vi "诊断标定4.vi"(8 "CAN端口":u16(ring), 9 "设备索引号":u16(ring), 10 "CAN卡类型":u32(ring)=4) -> ()   [LabVIEW 2013] (continued)
      n52 = property class="MCListbox (严格)"(reference=w20, "ItemNames"=w19) -> ()  [unwired: 1 in, 2 out]
      n53 = property on="全部读取" class="Bool (严格)"("Visible"=w95) -> ()  [unwired: 2 in, 2 out]
      n54 = Insert Into Array(array=w61, new element #1=w60, new element #2=w59, new element #3=w58, new element #4=w57, new element #5=w56) -> (w55:bool[])  [unwired: 1 in]
      n55 = local write "主从选择"(enum32{"主板", "从板"}."主板" ("主从选择")) -> ()
      n56 = And Array Elements(Boolean array=w55) -> (logical AND=w94:bool)
      n57 = property on="全部写入" class="Bool (严格)"("DisabledEnum"=2) -> ()  [unwired: 2 in, 2 out]
      n58 = local write "布尔"(w24) -> ()
      n59 = property on="全部写入" class="Bool (严格)"("Visible"=w94) -> ()  [unwired: 2 in, 2 out]
      n60 = local write "等级 2"(T13."从板信息" ("等级 2")) -> ()
      n61 = control-ref of="结果"() -> (w31:refnum<vi>)
      n62 = control-ref of="结果"() -> (w28:refnum<vi>)
      n63 = control-ref of="项目信息"() -> (w29:refnum<vi>)
      n64 = global write "EV05全局变量1.vi" "授权功能"(w25) -> ()
      n65 = local write "整车CAN测试"(w25) -> ()
      n66 = local write "判定2"(w25) -> ()
      n67 = local write "停止"(w25) -> ()
      n68 = local write "控制1"(w25) -> ()
      n69 = local write "消除"(w25) -> ()
      n70 = local write "继电器超时处理"(w25) -> ()
      n71 = local write "1 6"(w25) -> ()
      n72 = local write "1 7"(w25) -> ()
      n73 = local write "1 8"(w25) -> ()
      n74 = local write "1 9"(w25) -> ()
      n75 = local write "1 10"(w25) -> ()
      n76 = local write "1 2"(w25) -> ()
      n77 = local write "1 3"(w25) -> ()
      n78 = local write "1 4"(w25) -> ()
      n79 = local write "1 5"(w25) -> ()
      n80 = local write "1 11"(w25) -> ()
      n81 = local write "强制停止"(w25) -> ()
      n82 = for {
        N: 150 -> [_]
        tunnel: w31 -> [w123]
        i -> [w121]
        n83 = Bundle(w121, 0) -> (w119:cluster{i32, i32})  [unwired: 1 out]
        n84 = property class="MCListbox (严格)"(reference=w123, "ActiveCell"=w119, "CellBG"=u32 16448250) -> ()  [unwired: 1 in, 2 out]
        n85 = Wait Until Next ms Multiple(millisecond multiple=u32 1 ("毫秒倍数")) -> ()  [unwired: 1 out]
      }
      n86 = for {
        N: 150 -> [_]
        tunnel: w29 -> [w117]
        i -> [w116]
        n87 = Bundle(w116, 0) -> (w114:cluster{i32, i32})  [unwired: 1 out]
        n88 = property class="Tbl (严格)"(reference=w117, "Active Cell"=w114, "Cell BG Color"=u32 16448250) -> ()  [unwired: 1 in, 2 out]
        n89 = Wait Until Next ms Multiple(millisecond multiple=u32 1 ("毫秒倍数")) -> ()  [unwired: 1 out]
      }
      n90 = for {
        N: 150 -> [_]
        tunnel: w28 -> [w129]
        i -> [w127]
        n91 = Bundle(w127, 0) -> (w125:cluster{i32, i32})  [unwired: 1 out]
        n92 = property class="MCListbox (严格)"(reference=w129, "ActiveCell"=w125, "CellBG"=u32 16448250) -> ()  [unwired: 1 in, 2 out]
        n93 = Wait Until Next ms Multiple(millisecond multiple=u32 1 ("毫秒倍数")) -> ()  [unwired: 1 out]
      }
      n94 = stacked-sequence {
        tunnel: [w96 _] -> w23
        frame #0 {
          w103 = u8 0 items=["Normal", "Listen Only"] ("工作方式")
          w102 = u8 1 items=["Dual Filter", "Single Filter"] ("滤波方式")
          n95 = local read "设备索引号"() -> (w98:u16)
          n96 = local read "CAN卡类型"() -> (w97:u32)
          n97 = local read "CAN端口"() -> (w99:u16)
          n98 = call "CAN_Init-8.6.vi"("CAN卡类型"=w97, "设备索引号"=w98, "CAN端口"=w99, "操作类型"=enum16{"初始化CAN", "关闭CAN"}."初始化CAN", "滤波方式"=w102, "Accept Code"=u32 3221225472, "簇"=T20 {"打开CAN"=FALSE, "初始化CAN"=TRUE, "开始CAN"=TRUE, "重启"=FALSE, "关闭CAN"=FALSE}, "Mask Code"=u32 1073741823 ("Accept Code"), "工作方式"=w103, "是否滤波"=TRUE, "滤波选择"=T19 {"fiter_mode"=1, "fiter_endid"=402653184, "fiter_startid"=419430399}) -> ("error out"=w96:errorcluster)  [unwired: 3 in, 5 out]
        }
        frame #1 {
          n99 = local read "设备索引号"() -> (w109:u16)
          n100 = local read "CAN卡类型"() -> (w108:u32)
          n101 = local read "CAN端口"() -> (w110:u16)
          n102 = dll-call lib="PTH1Aabs EEV05EV05监控上位机-EV05EV05data\nusbcan.dll" fn="VCI_ClearBuffer"("DeviceType"=w108, "DeviceInd"=w109, "CANInd"=w110) -> (error out=w111:errorcluster)  [unwired: 4 in, 4 out]
          n103 = call <vilib>:"Clear Errors.vi"("error in (no error)"=w111) -> ()  [unwired: 6 in, 1 out]
        }
      }
      n104 = property on="保存版本信息" class="Bool (严格)"("Visible"=w25) -> ()  [unwired: 2 in, 2 out]
      n105 = local write "正级继电器"(w25) -> ()
      n106 = local write "负级继电器"(w25) -> ()
      n107 = local write "预充电继电器"(w25) -> ()
      n108 = local write "加热继电器"(w25) -> ()
      n109 = local write "充电继电器"(w25) -> ()
      n110 = local write "风机继电器"(w25) -> ()
      n111 = local write "加热继电器"(w25) -> ()
      n112 = local write "风机继电器"(w25) -> ()
      n113 = local write "DO1"(w25) -> ()
      n114 = local write "DO2"(w25) -> ()
      n115 = local write "DO1 2"(w25) -> ()
      n116 = local write "正级继电器 12"(w25) -> ()
      n117 = local write "正级继电器 2"(w25) -> ()
      n118 = local write "正级继电器 3"(w25) -> ()
      n119 = local write "正级继电器 4"(w25) -> ()
      n120 = local write "正级继电器 5"(w25) -> ()
      n121 = local write "正级继电器 6"(w25) -> ()
      n122 = local write "正级继电器 7"(w25) -> ()
      n123 = local write "正级继电器 8"(w25) -> ()
      n124 = local write "正级继电器 9"(w25) -> ()
      n125 = local write "正级继电器 10"(w25) -> ()
      n126 = local write "正级继电器 11"(w25) -> ()
      "电池故障" <- string[][] []
      "模块版本值" <- w36
      "硬件版本" <- w37
      "模块版本名称" <- w36
      "平台软件版本" <- w37
      "项目软件版本" <- w37
      "模块个数" <- u8[] [0, 0, 0, 0, 0, 0, 0, 0, 0, 0, 0, 0, 0, 0, 0, 0, 0, 0, 0, 0, 0, 0, 0, 0, 0, 0, 0, 0, 0, 0, 0, 0] ("模块个数")
      "单选选项2" <- w25
    }
  }
  n127 = stacked-sequence {
    frame #0 {
      n128 = control-ref of="从板选项"() -> (w132:refnum<vi>)
      n129 = stacked-sequence {
        tunnel: w132 -> [w135 w177 w212]
        frame #0 {
          n130 = global read "功能码全局.vi" "15"() -> (w159:bool[])
          n131 = global read "功能码全局.vi" "16"() -> (w150:bool[])
          n132 = Index Array(array=w159) -> (element #1=w158:bool, element #2=w156:bool, element #3=w154:bool, element #4=w152:bool, element #5=w157:bool, element #6=w155:bool, element #7=w153:bool, element #8=w151:bool)  [unwired: 8 in]
          n133 = Index Array(array=w150) -> (element #5=w141:bool, element #6=w149:bool, element #7=w140:bool, element #8=w148:bool)  [unwired: 8 in, 4 out]
          n134 = Not Or(1:w148, 2:w149) -> (0:w137:bool)
          n135 = Not Or(1:w140, 2:w141) -> (0:w139:bool)
          n136 = Not Or(1:w157, 2:w158) -> (0:w144:bool)
          n137 = Not Or(1:w155, 2:w156) -> (0:w145:bool)
          n138 = Not Or(1:w153, 2:w154) -> (0:w146:bool)
          n139 = Not Or(1:w151, 2:w152) -> (0:w147:bool)
          n140 = Compound Arithmetic op=OR(w144, w145, w146, w147, w137) -> (w143:bool)
          n141 = property class="Tree (严格)"(reference=w135, "Active Item Row Number"=1 ("活动项:行数"), "Disabled?"=w143, "Active Item Row Number"=2 ("活动项:行数"), "Disabled?"=w144, "Active Item Row Number"=3 ("活动项:行数"), "Disabled?"=w145, "Active Item Row Number"=4 ("活动项:行数"), "Disabled?"=w146, "Active Item Row Number"=5 ("活动项:行数"), "Disabled?"=w147, "Active Item Row Number"=0 ("活动项:行数"), "Disabled?"=w139) -> (error out=w134:errorcluster)  [unwired: 1 in, 1 out]
          n142 = for {
            N: 8 -> [_]
            tunnel: w135 -> [w171]
            tunnel: w137 -> [w167]
            tunnel: w134 -> [w166]
            tunnel: [w165] -> w138
            i -> [w169]
            n143 = Add(x=w169, y=6) -> (x+y=w170:i32)
            n144 = property class="Tree (严格)"(reference=w171, error in=w166, "Active Item Row Number"=w170, "Disabled?"=w167) -> (error out=w165:errorcluster)  [unwired: 1 out]
          }
          n145 = call <vilib>:"Clear Errors.vi"("error in (no error)"=w138) -> ()  [unwired: 6 in, 1 out]
        }
        frame #1 {
          w178 = 8
          n146 = global read "功能码全局.vi" "18"() -> (w187:bool[])
          n147 = Index Array(array=w187) -> (element #3=w186:bool, element #4=w181:bool, element #5=w174:bool, element #6=w185:bool, element #7=w180:bool, element #8=w173:bool)  [unwired: 8 in, 2 out]
          n148 = Not Or(1:w173, 2:w174) -> (0:w172:bool)
          n149 = Not Or(1:w185, 2:w186) -> (0:w184:bool)
          n150 = Not Or(1:w180, 2:w181) -> (0:w179:bool)
          n151 = for {
            N: w178 -> [_]
            tunnel: w177 -> [w208]
            tunnel: w184 -> [w204]
            tunnel: "error out" -> [w203]
            tunnel: [w202] -> w182
            i -> [w206]
            n152 = Add(x=w206, y=14) -> (x+y=w207:i32)
            n153 = property class="Tree (严格)"(reference=w208, error in=w203, "Active Item Row Number"=w207, "Disabled?"=w204) -> (error out=w202:errorcluster)  [unwired: 1 out]
          }
          n154 = for {
            N: w178 -> [_]
            tunnel: w177 -> [w201]
            tunnel: w179 -> [w197]
            tunnel: w182 -> [w196]
            tunnel: [w195] -> w176
            i -> [w199]
            n155 = Add(x=w199, y=22) -> (x+y=w200:i32)
            n156 = property class="Tree (严格)"(reference=w201, error in=w196, "Active Item Row Number"=w200, "Disabled?"=w197) -> (error out=w195:errorcluster)  [unwired: 1 out]
          }
          n157 = for {
            N: w178 -> [_]
            tunnel: w177 -> [w194]
            tunnel: w172 -> [w190]
            tunnel: w176 -> [w189]
            tunnel: [w188] -> w175
            i -> [w192]
            n158 = Add(x=w192, y=30) -> (x+y=w193:i32)
            n159 = property class="Tree (严格)"(reference=w194, error in=w189, "Active Item Row Number"=w193, "Disabled?"=w190) -> (error out=w188:errorcluster)  [unwired: 1 out]
          }
          n160 = call <vilib>:"Clear Errors.vi"("error in (no error)"=w175) -> ()  [unwired: 6 in, 1 out]
        }
        frame #2 {
          n161 = for {
            N: 8 -> [_]
            tunnel: w212 -> [w220]
            tunnel: TRUE -> [w216]
            tunnel: errorcluster {"status"=FALSE, "code"=0, "source"=""} ("error out 2") -> [w215]
            tunnel: [w214] -> w211
            i -> [w218]
            n162 = Add(x=w218, y=38) -> (x+y=w219:i32)
            n163 = property class="Tree (严格)"(reference=w220, error in=w215, "Active Item Row Number"=w219, "Disabled?"=w216) -> (error out=w214:errorcluster)  [unwired: 1 out]
          }
          n164 = call <vilib>:"Clear Errors.vi"("error in (no error)"=w211) -> ()  [unwired: 6 in, 1 out]
        }
      }
      n165 = control-ref of="主板选项"() -> (w133:refnum<vi>)
      n166 = stacked-sequence {
        tunnel: w133 -> [w250 w288 w338]
        frame #0 {
          # "项目信息"
          # "SOC"
          # "SOH"
          # "电池额定实际容量"
          # "车牌号"
          # "产品编号"
          # "电压个数"
          # "通道电压数"
          # "温度个数"
          # "电压起始值"
          # "温度起始值"
          # "配置文件版本"
          # "系统时钟"
          # "校正时钟"
          n167 = global read "功能码全局.vi" "主板项目信息5"() -> (w283:bool[])
          n168 = global read "功能码全局.vi" "主板项目信息6"() -> (w282:bool[])
          n169 = global read "功能码全局.vi" "主板项目信息7"() -> (w259:bool[])
          n170 = global read "功能码全局.vi" "主板项目信息4"() -> (w230:bool[])
          n171 = global read "功能码全局.vi" "主板监控2"() -> (w221:bool[])
          n172 = Index Array(array=w283) -> (element #1=w280:bool, element #2=w277:bool, element #3=w274:bool, element #4=w271:bool, element #5=w267:bool, element #6=w265:bool, element #7=w262:bool, element #8=w258:bool)  [unwired: 8 in]
          n173 = Index Array(array=w282) -> (element #1=w255:bool, element #2=w279:bool, element #3=w276:bool, element #4=w273:bool, element #5=w270:bool, element #6=w266:bool, element #7=w264:bool, element #8=w261:bool)  [unwired: 8 in]
          n174 = Index Array(array=w259) -> (element #1=w257:bool, element #2=w254:bool, element #3=w252:bool, element #4=w247:bool, element #5=w244:bool, element #6=w251:bool, element #7=w245:bool, element #8=w243:bool)  [unwired: 8 in]
          n175 = Index Array(array=w221) -> (element #8=w222:bool)  [unwired: 8 in, 7 out]
          n176 = Index Array(array=w230) -> (element #6=w226:bool, element #7=w225:bool, element #8=w229:bool)  [unwired: 8 in, 5 out]
          n177 = property on="读配置文件" class="Bool (严格)"("Visible"=w222) -> ()  [unwired: 2 in, 2 out]
          n178 = Not(x=w229) -> (.not. x?=w228:bool)
          n179 = Not Or(1:w225, 2:w226) -> (0:w224:bool)
          n180 = Not Or(1:w279, 2:w280) -> (0:w242:bool)
          n181 = Not Or(1:w276, 2:w277) -> (0:w241:bool)
          n182 = Not Or(1:w273, 2:w274) -> (0:w240:bool)
          n183 = Not Or(1:w270, 2:w271) -> (0:w239:bool)
          n184 = Not Or(1:w266, 2:w267) -> (0:w238:bool)
          n185 = Not Or(1:w264, 2:w265) -> (0:w237:bool)
          n186 = Not Or(1:w261, 2:w262) -> (0:w236:bool)
          n187 = Not Or(1:w257, 2:w258) -> (0:w235:bool)
          n188 = Not Or(1:w251, 2:w252) -> (0:w233:bool)
          n189 = Not Or(1:w243, 2:w244) -> (0:w231:bool)
          n190 = Not Or(1:w245, 2:w247) -> (0:w232:bool)
          n191 = Not Or(1:w254, 2:w255) -> (0:w234:bool)
          n192 = Compound Arithmetic op=OR(w228, w242, w241, w240, w239, w238, w237, w236, w235, w234, w233, w232, w231) -> (w223:bool)
          n193 = property class="Tree (严格)"(reference=w250, "Active Item Row Number"=9 ("活动项:行数"), "Disabled?"=w224, "Active Item Row Number"=1 ("活动项:行数"), "Disabled?"=w223, "Active Item Row Number"=0 ("活动项:行数"), "Disabled?"=w228, "Active Item Row Number"=3 ("活动项:行数"), "Disabled?"=w242, "Active Item Row Number"=4 ("活动项:行数"), "Disabled?"=w241, "Active Item Row Number"=5 ("活动项:行数"), "Disabled?"=w240, "Active Item Row Number"=6 ("活动项:行数"), "Disabled?"=w239, "Active Item Row Number"=7 ("活动项:行数"), "Disabled?"=w238, "Active Item Row Number"=8 ("活动项:行数"), "Disabled?"=w237, "Active Item Row Number"=11 ("活动项:行数"), "Disabled?"=w236, "Active Item Row Number"=12 ("活动项:行数"), "Disabled?"=w235, "Active Item Row Number"=13 ("活动项:行数"), "Disabled?"=w234, "Active Item Row Number"=2 ("活动项:行数"), "Disabled?"=w233, "Active Item Row Number"=10 ("活动项:行数"), "Disabled?"=w232, "Active Item Row Number"=14 ("活动项:行数"), "Disabled?"=w231) -> ()  [unwired: 1 in, 2 out]
        }
        frame #1 {
          w293 = 18
          # "一二三级故障"
          n194 = global read "功能码全局.vi" "主板故障阀值9"() -> (w299:bool[])
          n195 = Index Array(array=w299) -> (element #3=w298:bool, element #4=w295:bool, element #5=w292:bool, element #6=w297:bool, element #7=w294:bool, element #8=w291:bool)  [unwired: 8 in, 2 out]
          n196 = Not Or(1:w297, 2:w298) -> (0:w287:bool)
          n197 = Not Or(1:w294, 2:w295) -> (0:w285:bool)
          n198 = Not Or(1:w291, 2:w292) -> (0:w286:bool)
          n199 = for {
            N: w293 -> [_]
            tunnel: w288 -> [w319]
            tunnel: w287 -> [w315]
            tunnel: [w314] -> w296
            i -> [w317]
            n200 = Add(x=w317, y=15) -> (x+y=w318:i32)
            n201 = property class="Tree (严格)"(reference=w319, "Active Item Row Number"=w318, "Disabled?"=w315) -> (error out=w314:errorcluster)  [unwired: 1 in, 1 out]
          }
          n202 = for {
            N: w293 -> [_]
            tunnel: w288 -> [w313]
            tunnel: w285 -> [w309]
            tunnel: w296 -> [w308]
            tunnel: [w307] -> w290
            i -> [w311]
            n203 = Add(x=w311, y=33) -> (x+y=w312:i32)
            n204 = property class="Tree (严格)"(reference=w313, error in=w308, "Active Item Row Number"=w312, "Disabled?"=w309) -> (error out=w307:errorcluster)  [unwired: 1 out]
          }
          n205 = for {
            N: w293 -> [_]
            tunnel: w288 -> [w306]
            tunnel: w286 -> [w302]
            tunnel: w290 -> [w301]
            tunnel: [w300] -> w289
            i -> [w304]
            n206 = Add(x=w304, y=51) -> (x+y=w305:i32)
            n207 = property class="Tree (严格)"(reference=w306, error in=w301, "Active Item Row Number"=w305, "Disabled?"=w302) -> (error out=w300:errorcluster)  [unwired: 1 out]
          }
          n208 = call <vilib>:"Clear Errors.vi"("error in (no error)"=w289) -> ()  [unwired: 6 in, 1 out]
        }
        frame #2 {
          # "电池信息"
          # "加热和充电控制参数"
          n209 = global read "功能码全局.vi" "主板版本号11"() -> (w339:bool[])
          n210 = global read "功能码全局.vi" "主板控制类信息10"() -> (w349:bool[])
          n211 = Index Array(array=w339) -> (element #1=w335:bool, element #2=w334:bool, element #3=w327:bool, element #4=w326:bool, element #6=w323:bool, element #7=w322:bool, element #8=w321:bool)  [unwired: 8 in, 1 out]
          n212 = control-ref of="单选选项2"() -> (w328:refnum<vi>)
          n213 = Or(x=w327, y=w326) -> (x .or. y?=w325:bool)
          n214 = Index Array(array=w349) -> (element #5=w343:bool, element #6=w341:bool, element #7=w342:bool, element #8=w340:bool)  [unwired: 8 in, 4 out]
          n215 = property class="Bool (严格)"(reference=w328, "Visible"=w325) -> ()  [unwired: 1 in, 2 out]
          n216 = Not(x=w322) -> (.not. x?=w330:bool)
          n217 = Not(x=w321) -> (.not. x?=w329:bool)
          n218 = Not(x=w323) -> (.not. x?=w331:bool)
          n219 = property on="硬件版本号" class="Str"("Visible"=w327) -> ()  [unwired: 2 in, 2 out]
          n220 = property on="读硬件版本号" class="Bool (严格)"("Visible"=w327) -> ()  [unwired: 2 in, 2 out]
          n221 = property on="项目软件版本号" class="Str"("Visible"=w327) -> ()  [unwired: 2 in, 2 out]
          n222 = property on="项目软本读取" class="Bool (严格)"("Visible"=w327) -> ()  [unwired: 2 in, 2 out]
          n223 = property on="继电器屏1" class="TabCtl (严格)"("Visible"=w331) -> ()  [unwired: 2 in, 2 out]
          n224 = property on="均衡屏" class="TabCtl (严格)"("Visible"=w329) -> ()  [unwired: 2 in, 2 out]
          n225 = property on="继电器屏1 2" class="TabCtl (严格)"("Visible"=w331) -> ()  [unwired: 2 in, 2 out]
          n226 = property on="DO屏" class="TabCtl (严格)"("Visible"=w330) -> ()  [unwired: 2 in, 2 out]
          n227 = Not Or(1:w342, 2:w343) -> (0:w348:bool)
          n228 = Not Or(1:w340, 2:w341) -> (0:w346:bool)
          n229 = Not Or(1:w334, 2:w335) -> (0:w333:bool)
          n230 = for {
            N: 8 -> [_]
            tunnel: w338 -> [w369]
            tunnel: w348 -> [w365]
            tunnel: [w364] -> w347
            i -> [w367]
            n231 = Add(x=w367, y=69) -> (x+y=w368:i32)
            n232 = property class="Tree (严格)"(reference=w369, "Active Item Row Number"=w368, "Disabled?"=w365) -> (error out=w364:errorcluster)  [unwired: 1 in, 1 out]
          }
          n233 = for {
            N: 9 -> [_]
            tunnel: w338 -> [w363]
            tunnel: w346 -> [w359]
            tunnel: w347 -> [w358]
            tunnel: [w357] -> w337
            i -> [w361]
            n234 = Add(x=w361, y=77) -> (x+y=w362:i32)
            n235 = property class="Tree (严格)"(reference=w363, error in=w358, "Active Item Row Number"=w362, "Disabled?"=w359) -> (error out=w357:errorcluster)  [unwired: 1 out]
          }
          n236 = for {
            N: 5 -> [_]
            tunnel: w338 -> [w356]
            tunnel: w333 -> [w352]
            tunnel: w337 -> [w351]
            tunnel: [w350] -> w336
            i -> [w354]
            n237 = Add(x=w354, y=86) -> (x+y=w355:i32)
            n238 = property class="Tree (严格)"(reference=w356, error in=w351, "Active Item Row Number"=w355, "Disabled?"=w352) -> (error out=w350:errorcluster)  [unwired: 1 out]
          }
          n239 = Compound Arithmetic op=OR(w323, w322, w321) -> (w320:bool)
          n240 = property on="模块软件版本" class="MCListbox (严格)"("Visible"=w326) -> ()  [unwired: 2 in, 2 out]
          n241 = property on="模块软件版本" class="Enum (严格)"("Visible"=w326) -> ()  [unwired: 2 in, 2 out]
          n242 = property on="平台软件版本号" class="Str"("Visible"=w326) -> ()  [unwired: 2 in, 2 out]
          n243 = control-ref of="单选选项2 2"() -> (w324:refnum<vi>)
          n244 = property class="Bool (严格)"(reference=w324, "Visible"=w320) -> ()  [unwired: 1 in, 2 out]
          n245 = property on="模块版本读取" class="Bool (严格)"("Visible"=w326) -> ()  [unwired: 2 in, 2 out]
          n246 = property on="平台软件版本读取" class="Bool (严格)"("Visible"=w326) -> ()  [unwired: 2 in, 2 out]
          n247 = call <vilib>:"Clear Errors.vi"("error in (no error)"=w336) -> ()  [unwired: 6 in, 1 out]
        }
      }
    }
  }
  n248 = call "自适应屏幕分辨率.vi"() -> ()  [unwired: 16 in]
  n249 = Obtain Queue(name (unnamed)=w18, element data type=w18) -> (queue out=w17:refnum<queue>, error out=w16:errorcluster)  [unwired: 3 in, 1 out]
  n250 = Obtain Queue(element data type="输出簇") -> (queue out=w11:refnum<queue>, error out=w10:errorcluster)  [unwired: 4 in, 1 out]
  n251 = while {
    tunnel: w17 -> [w373]
    tunnel: w16 -> [w372]
    stop <- w370 stop-if-true
    n252 = Dequeue Element(queue=w373, error in (no error)=w372) -> (element=w371:string, error out=w370:errorcluster)  [unwired: 3 out]
    n253 = case shown="无错误" w370 {
      tunnel: w371 -> [w374 _]
      frame No Error {
        n254 = case shown="\"开启均衡\"" w374 {
          frame "假", Default {
          }
          frame "单个写入" {
            n255 = local read "主从选择"() -> (w381:enum32{"主板", "从板"})
            n256 = case shown="\"从板\"" w381 {
              tunnel: [w392 w407] -> w378
              tunnel: [0.0 w405] -> w382
              tunnel: [_ w406] -> w380
              tunnel: [w390 _] -> w379
              frame "主板", Default {
                n257 = stacked-sequence {
                  tunnel: [_ w404] -> w390
                  frame #0 {
                    n258 = control-ref of="高压参数"() -> (w395:refnum<vi>)
                    n259 = control-ref of="电池信息"() -> (w396:refnum<vi>)
                    n260 = control-ref of="一级故障"() -> (w402:refnum<vi>)
                    n261 = control-ref of="一级故障 2"() -> (w400:refnum<vi>)
                    n262 = control-ref of="一级故障 3"() -> (w399:refnum<vi>)
                    n263 = control-ref of="加热控制参数"() -> (w398:refnum<vi>)
                    n264 = control-ref of="充电控制参数"() -> (w397:refnum<vi>)
                    n265 = control-ref of="项目信息"() -> (w401:refnum<vi>)
                    n266 = control-ref of="一级故障 4"() -> (w403:refnum<vi>)
                    n267 = local read "主板数据"() -> (w393:T4)
                    n268 = Bundle(cluster=w393, "项目信息"=w401, "一级故障 4"=w403, "一级故障"=w402, "一级故障 2"=w400, "一级故障 3"=w399, "加热控制参数"=w398, "充电控制参数"=w397, "高压参数"=w395, "电池信息"=w396) -> (w394:T4)
                    n269 = local write "主板数据"(w394) -> ()
                  }
                  frame #1 {
                    n270 = control-ref of="主板数据"() -> (w404:refnum<vi>)
                  }
                }
                n271 = local read "主板选项"() -> (w392:string)
              }
              frame "从板" {
                n272 = stacked-sequence {
                  tunnel: [_ w416] -> w406
                  frame #0 {
                    n273 = control-ref of="从板板号"() -> (w415:refnum<vi>)
                    n274 = control-ref of="项目信息 2"() -> (w414:refnum<vi>)
                    n275 = control-ref of="加热控制参数"() -> (w413:refnum<vi>)
                    n276 = control-ref of="一级故障(从板)"() -> (w412:refnum<vi>)
                    n277 = control-ref of="二级故障(从板)"() -> (w411:refnum<vi>)
                    n278 = control-ref of="三级故障(从板)"() -> (w410:refnum<vi>)
                    n279 = control-ref of="电池组信息(从板)"() -> (w409:refnum<vi>)
                    n280 = Bundle("从板板号"=w415, "项目信息 2"=w414, "加热控制参数"=w413, "一级故障(从板)"=w412, "二级故障(从板)"=w411, "三级故障(从板)"=w410, "电池组信息(从板)"=w409) -> (w408:T3)  [unwired: 1 in]
                    n281 = local write "从板数据"(w408) -> ()
                  }
                  frame #1 {
                    n282 = control-ref of="从板数据"() -> (w416:refnum<vi>)
                  }
                }
                n283 = local read "从板选项"() -> (w407:string)
                n284 = local read "从板板号"() -> (w405:u8)
              }
            }
            n285 = local read "从板个数"() -> (w383:dbl)
            n286 = local read "快换"() -> (w384:bool)
            n287 = call "输入数据解析.vi"("单个参数补充"=w383, "从板号"=w382, "主板引用"=w379, "从板引用"=w380, "主板选项"=w378, "枚举"=w381, "快换"=w384) -> ("输出数组"=w388:dbl[][], "数组长度"=w387:dbl[], "循环次数"=w377:i32, "命令"=w386:u32, "名称"=w376:string[], "命令序号"=w385:u32[])  [unwired: 3 out]
            n288 = for {
              N: w377 -> [w422]
              tunnel: w388 -> [w432]
              tunnel: w387 -> [w431]
              tunnel: w386 -> [w430]
              tunnel: w385 -> [w429]
              tunnel: w382 -> [w420]
              tunnel: w378 -> [w428]
              tunnel: w376 -> [w424]
              tunnel: [w417] -> w375
              i -> [w423]
              n289 = Index Array(array=w432, index (row)=w423) -> (element=w427:dbl[])  [unwired: 1 in]
              n290 = Index Array(array=w424, index=w423) -> (element=w421:string)
              n291 = case shown="\"从板号\"" w421 {
                tunnel: [w434 w435] -> w419
                tunnel: w420 -> [w434 _]
                tunnel: [TRUE ("确定") w436] -> w418
                frame "假", Default {
                }
                frame "从板号" {
                  n292 = call "请输入当前从板板号"() -> ("当前从板板号"=w435:dbl, "确定"=w436:bool)  [unwired: 17 in, 1 out]
                  n293 = local write "当前从板板号"(w435) -> ()
                }
              }
              n294 = Index Array(array=w429, index=w423) -> (element=w425:u32)
              n295 = Index Array(array=w431, index=w423) -> (element=w426:dbl)
              n296 = global write "全局 1.vi" "名称"(w421) -> ()
              n297 = case shown="真" w418 {
                tunnel: w430 -> [_ w446]
                tunnel: w428 -> [_ w445]
                tunnel: w427 -> [_ w444]
                tunnel: w426 -> [_ w443]
                tunnel: w425 -> [_ w442]
                tunnel: w423 -> [_ w441]
                tunnel: w421 -> [_ w440]
                tunnel: w422 -> [_ w439]
                tunnel: w419 -> [_ w438]
                tunnel: [_ w437] -> w417
                frame False {
                  n298 = call <vilib>:"Unset Busy.vi"() -> ()  [unwired: 11 in, 1 out]
                }
                frame True {
                  n299 = stacked-sequence {
                    seq-local: [_ _ w475 _ _] -> [_ _ _ w484 _]
                    tunnel: w444 -> [_ w463 _ _ _]
                    tunnel: w443 -> [_ w462 _ _ _]
                    tunnel: w446 -> [_ w456 _ _ _]
                    tunnel: w442 -> [_ w454 _ _ _]
                    tunnel: w445 -> [_ _ _ _ _]
                    tunnel: w441 -> [_ _ _ _ w495]
                    tunnel: w440 -> [_ _ _ w483 _]
                    tunnel: w439 -> [_ _ _ _ w496]
                    tunnel: w438 -> [_ w455 _ _ _]
                    tunnel: [_ _ _ _ w493] -> w437
                    frame #0 {
                      n300 = global write "EV05全局变量1.vi" "读取超时"(FALSE ("读取超时")) -> ()
                      n301 = local write "消除"(TRUE ("消除")) -> ()
                      n302 = call <vilib>:"Set Busy.vi"("disable click? (T)"=FALSE) -> ()  [unwired: 3 in, 8 out]
                      n303 = global write "EV05全局变量1.vi" "流控帧 2"(FALSE ("流控帧 2")) -> ()
                      n304 = local write "控制1"(TRUE ("控制1")) -> ()
                      n305 = local write "写?"(TRUE ("写?")) -> ()
                      n306 = Wait Until Next ms Multiple(millisecond multiple=u32 50 ("毫秒倍数")) -> ()  [unwired: 1 out]
                    }
                    frame #1 {
                      n307 = local read "设备索引号"() -> (w458:u16)
                      n308 = local read "CAN卡类型"() -> (w459:u32)
                      n309 = Increment(x=w462) -> (x+1=w461:dbl)
                      n310 = local read "CAN端口"() -> (w457:u16)
                      n311 = local write "命令"(w456) -> ()
                      n312 = local write "命令序号"(w454) -> ()
                      n313 = Reshape Array(w463, w461) -> (w460:dbl[])
                      n314 = stacked-sequence {
                        tunnel: w460 -> [_ w474]
                        tunnel: w459 -> [w466 w473]
                        tunnel: w458 -> [w465 w472]
                        tunnel: w457 -> [w464 w471]
                        tunnel: w456 -> [_ w470]
                        tunnel: w455 -> [_ w469]
                        tunnel: w454 -> [_ w468]
                        frame #0 {
                          n315 = dll-call lib="PTH1Aabs EEV05EV05监控上位机-EV05EV05data\nusbcan.dll" fn="VCI_ClearBuffer"("DeviceType"=w466, "DeviceInd"=w465, "CANInd"=w464) -> (error out=w467:errorcluster)  [unwired: 4 in, 4 out]
                          n316 = call <vilib>:"Clear Errors.vi"("error in (no error)"=w467) -> ()  [unwired: 6 in, 1 out]
                        }
                        frame #1 {
                          n317 = call "多帧发送机制(EV05).vi"("can卡类型"=w473, "设备索引号"=w472, "CAN端口"=w471, "命令"=w470, "板号"=w469, "命令序号"=w468, "输入数据"=w474) -> ()  [unwired: 1 in, 12 out]
                        }
                      }
                    }
                    frame #2 {
                      n318 = while {
                        tunnel: [w477] -> w475
                        i -> [w481]
                        stop <- w478 stop-if-true
                        n319 = global read "EV05全局变量1.vi" "读取超时"() -> (w477:bool)
                        n320 = local read "强制停止"() -> (w476:bool)
                        n321 = Greater Or Equal?(x=w481, y=25) -> (x >= y?=w479:bool)
                        n322 = Wait Until Next ms Multiple(millisecond multiple=u32 100 ("毫秒倍数")) -> ()  [unwired: 1 out]
                        n323 = Compound Arithmetic op=OR(w476, w477, w479) -> (w478:bool)
                      }
                    }
                    frame #3 {
                      n324 = case shown="假" w484 {
                        tunnel: w483 -> [w485 w491]
                        frame False {
                          n325 = control-ref of="结果"() -> (w489:refnum<vi>)
                          n326 = Concatenate Strings(w485, "       写入失败" ("字符串")) -> (w488:string)
                          n327 = Build Array(w488) -> (w487:string[])
                          n328 = call "表格编辑.vi"("新元素/子数组"=w487, "活动单元格:单元格背景色"=u32 16740749, "MCListbox引用句柄"=w489) -> ()  [unwired: 9 out]
                        }
                        frame True {
                          n329 = case shown="\"从板号\"" w491 {
                            frame "假", Default {
                            }
                            frame "从板号" {
                              n330 = local read "从板板号"() -> (w492:u8)
                              n331 = local write "当前从板板号"(w492) -> ()
                            }
                          }
                        }
                      }
                      n332 = call <vilib>:"Unset Busy.vi"() -> ()  [unwired: 2 in, 10 out]
                    }
                    frame #4 {
                      n333 = Increment(x=w495) -> (x+1=w494:i32)
                      n334 = Equal?(x=w496, y=w494) -> (x = y?=w493:bool)
                      n335 = case shown="真" w493 {
                        frame False {
                        }
                        frame True {
                          n336 = control-ref of="结果"() -> (w500:refnum<vi>)
                          n337 = Concatenate Strings("写入完成" ("字符串")) -> (w499:string)
                          n338 = Build Array(w499) -> (w498:string[])
                          n339 = call "表格编辑.vi"("新元素/子数组"=w498, "活动单元格:单元格背景色"=u32 21937, "MCListbox引用句柄"=w500) -> ()  [unwired: 9 out]
                        }
                      }
                    }
                  }
                }
              }
            }
            n340 = stacked-sequence {
              tunnel: w375 -> [_]
              frame #0 {
                n341 = local write "强制停止"(FALSE ("强制停止")) -> ()
              }
            }
          }
          frame "全部写入" {
            n342 = local read "主从选择"() -> (w507:enum32{"主板", "从板"})
            n343 = case shown="\"主板\", 默认" w507 {
              tunnel: [string[] ["项目信息", "一级故障阀值", "二级故障阀值", "三级故障阀值", "加热控制参数", "充电控制参数", "电池信息"] string[] ["从板信息", "一级故障阀值", "二级故障阀值", "三级故障阀值"]] -> w504
              tunnel: [0.0 ("从板号") w642] -> w508
              tunnel: [w627 _] -> w506
              tunnel: [_ w643] -> w505
              frame "主板", Default {
                n344 = stacked-sequence {
                  tunnel: [_ w641] -> w627
                  frame #0 {
                    n345 = control-ref of="电池信息"() -> (w633:refnum<vi>)
                    n346 = control-ref of="高压参数"() -> (w632:refnum<vi>)
                    n347 = control-ref of="一级故障"() -> (w635:refnum<vi>)
                    n348 = control-ref of="一级故障 2"() -> (w637:refnum<vi>)
                    n349 = control-ref of="一级故障 3"() -> (w638:refnum<vi>)
                    n350 = control-ref of="加热控制参数"() -> (w639:refnum<vi>)
                    n351 = control-ref of="充电控制参数"() -> (w640:refnum<vi>)
                    n352 = control-ref of="项目信息"() -> (w636:refnum<vi>)
                    n353 = control-ref of="一级故障 4"() -> (w634:refnum<vi>)
                    n354 = local read "主板数据"() -> (w631:T4)
                    n355 = Bundle(cluster=w631, "项目信息"=w636, "一级故障 4"=w634, "一级故障"=w635, "一级故障 2"=w637, "一级故障 3"=w638, "加热控制参数"=w639, "充电控制参数"=w640, "高压参数"=w632, "电池信息"=w633) -> (w630:T4)
                    n356 = local write "主板数据"(w630) -> ()
                  }
                  frame #1 {
                    n357 = control-ref of="主板数据"() -> (w641:refnum<vi>)
                  }
                }
              }
              frame "从板" {
                n358 = stacked-sequence {
                  tunnel: [_ w654] -> w643
                  frame #0 {
                    n359 = control-ref of="从板板号"() -> (w647:refnum<vi>)
                    n360 = control-ref of="项目信息 2"() -> (w648:refnum<vi>)
                    n361 = control-ref of="加热控制参数"() -> (w649:refnum<vi>)
                    n362 = control-ref of="一级故障(从板)"() -> (w650:refnum<vi>)
                    n363 = control-ref of="二级故障(从板)"() -> (w651:refnum<vi>)
                    n364 = control-ref of="三级故障(从板)"() -> (w652:refnum<vi>)
                    n365 = control-ref of="电池组信息(从板)"() -> (w653:refnum<vi>)
                    n366 = local read "从板数据"() -> (w645:T3)
                    n367 = Bundle(cluster=w645, "从板板号"=w647, "项目信息 2"=w648, "加热控制参数"=w649, "一级故障(从板)"=w650, "二级故障(从板)"=w651, "三级故障(从板)"=w652, "电池组信息(从板)"=w653) -> (w646:T3)
                    n368 = local write "从板数据"(w646) -> ()
                  }
                  frame #1 {
                    n369 = control-ref of="从板数据"() -> (w654:refnum<vi>)
                  }
                }
                n370 = local read "从板板号"() -> (w642:u8)
              }
            }
            n371 = Array Size(array=w504) -> (size(s)=w503:i32)
            n372 = while {
              tunnel: w504 -> [w516] mode=indexing
              tunnel: w507 -> [w520]
              tunnel: w508 -> [w523]
              tunnel: w506 -> [w522]
              tunnel: w505 -> [w521]
              tunnel: w503 -> [w514]
              tunnel: [w510] -> w502
              i -> [w515]
              stop <- w511 stop-if-true
              n373 = Increment(x=w515) -> (x+1=w513:i32)
              n374 = local read "从板个数"() -> (w528:dbl)
              n375 = local read "快换"() -> (w519:bool)
              n376 = Less Or Equal?(x=w514, y=w513) -> (x <= y?=w510:bool)
              n377 = call "输入数据解析.vi"("单个参数补充"=w528, "从板号"=w523, "主板引用"=w522, "从板引用"=w521, "主板选项"=w516, "枚举"=w520, "快换"=w519) -> ("输出数组"=w527:dbl[][], "数组长度"=w526:dbl[], "循环次数"=w518:i32, "命令"=w525:u32, "名称"=w517:string[], "命令序号"=w524:u32[])  [unwired: 3 out]
              n378 = case shown="\"从板\"" w520 {
                tunnel: w515 -> [w530 w544]
                frame "主板", Default {
                  n379 = case shown="6" w530 {
                    tunnel: [T7."项目信息" ("主从板") T7."一级故障阀值" ("主从板") T7."二级故障阀值" ("主从板") T7."三级故障阀值" ("主从板") T7."控制参数" ("主从板") T7."电池信息" ("主从板")] -> w529
                    frame 0, Default {
                      n380 = local write "1"(TRUE ("1")) -> ()
                    }
                    frame 1 {
                      n381 = local write "1 2"(TRUE ("1 2")) -> ()
                    }
                    frame 2 {
                      n382 = local write "1 3"(TRUE ("1 3")) -> ()
                    }
                    frame 3 {
                      n383 = local write "1 4"(TRUE ("1 4")) -> ()
                    }
                    frame 4, 5 {
                      n384 = local write "1 5"(TRUE ("1 5")) -> ()
                    }
                    frame 6 {
                      n385 = local write "1 11"(TRUE ("1 11")) -> ()
                    }
                  }
                  n386 = local write "主板2"(w529) -> ()
                }
                frame "从板" {
                  n387 = case shown="4" w544 {
                    tunnel: [T13."从板信息" ("等级 2") T13."从板信息" ("等级 2") T13."一级故障阀值" ("等级 2") T13."二级故障阀值" ("等级 2") T13."三级故障阀值" ("等级 2") T13."快换参数" ("等级 2")] -> w543
                    frame 99, Default {
                      n388 = local write "1 6"(TRUE ("1 6")) -> ()
                    }
                    frame 0 {
                      n389 = local write "1 6"(TRUE ("1 6")) -> ()
                    }
                    frame 1 {
                      n390 = local write "1 7"(TRUE ("1 7")) -> ()
                    }
                    frame 2 {
                      n391 = local write "1 8"(TRUE ("1 8")) -> ()
                    }
                    frame 3 {
                      n392 = local write "1 9"(TRUE ("1 9")) -> ()
                    }
                    frame 4 {
                      n393 = local write "1 10"(TRUE ("1 10")) -> ()
                    }
                  }
                  n394 = local write "等级 2"(w543) -> ()
                }
              }
              n395 = for {
                N: w518 -> [w559]
                tunnel: w527 -> [w569]
                tunnel: w526 -> [w568]
                tunnel: w525 -> [w567]
                tunnel: w524 -> [w565]
                tunnel: w523 -> [w566]
                tunnel: w517 -> [w562]
                tunnel: w510 -> [w557]
                i -> [w558]
                n396 = Index Array(array=w569, index (row)=w558) -> (element=w564:dbl[])  [unwired: 1 in]
                n397 = Index Array(array=w568, index=w558) -> (element=w563:dbl)
                n398 = Index Array(array=w562, index=w558) -> (element=w560:string)
                n399 = Index Array(array=w565, index=w558) -> (element=w561:u32)
                n400 = stacked-sequence {
                  seq-local: [_ _ w600 _ _] -> [_ _ _ w609 _]
                  tunnel: w564 -> [_ w584 _ _ _]
                  tunnel: w563 -> [_ w583 _ _ _]
                  tunnel: w567 -> [_ w578 _ _ _]
                  tunnel: w566 -> [_ w581 _ _ _]
                  tunnel: w561 -> [_ w579 _ _ _]
                  tunnel: w560 -> [_ w577 _ w608 _]
                  tunnel: w559 -> [_ _ _ _ w621]
                  tunnel: w558 -> [_ _ _ _ w620]
                  tunnel: w557 -> [_ _ _ _ w618]
                  frame #0 {
                    n401 = global write "EV05全局变量1.vi" "读取超时"(FALSE ("读取超时")) -> ()
                    n402 = global write "EV05全局变量1.vi" "流控帧 2"(FALSE ("流控帧 2")) -> ()
                    n403 = local write "写?"(TRUE ("写?")) -> ()
                    n404 = local write "控制1"(TRUE ("控制1")) -> ()
                    n405 = local write "消除"(TRUE ("消除")) -> ()
                    n406 = call <vilib>:"Set Busy.vi"("disable click? (T)"=FALSE) -> ()  [unwired: 3 in, 8 out]
                    n407 = Wait Until Next ms Multiple(millisecond multiple=u32 20 ("毫秒倍数")) -> ()  [unwired: 1 out]
                  }
                  frame #1 {
                    n408 = global write "全局 1.vi" "名称"(w577) -> ()
                    n409 = local write "命令序号"(w579) -> ()
                    n410 = local write "命令"(w578) -> ()
                    n411 = local read "设备索引号"() -> (w586:u16)
                    n412 = local read "CAN卡类型"() -> (w587:u32)
                    n413 = Increment(x=w583) -> (x+1=w580:dbl)
                    n414 = local read "CAN端口"() -> (w585:u16)
                    n415 = Reshape Array(w584, w580) -> (w582:dbl[])
                    n416 = stacked-sequence {
                      tunnel: w587 -> [w590 w599]
                      tunnel: w586 -> [w589 w598]
                      tunnel: w585 -> [w588 w597]
                      tunnel: w582 -> [_ w596]
                      tunnel: w581 -> [_ w595]
                      tunnel: w579 -> [_ w594]
                      tunnel: w578 -> [_ w593]
                      frame #0 {
                        n417 = dll-call lib="PTH1Aabs EEV05EV05监控上位机-EV05EV05data\nusbcan.dll" fn="VCI_ClearBuffer"("DeviceType"=w590, "DeviceInd"=w589, "CANInd"=w588) -> (error out=w591:errorcluster)  [unwired: 4 in, 4 out]
                        n418 = call <vilib>:"Clear Errors.vi"("error in (no error)"=w591) -> ()  [unwired: 6 in, 1 out]
                      }
                      frame #1 {
                        n419 = call "多帧发送机制(EV05).vi"("can卡类型"=w599, "设备索引号"=w598, "CAN端口"=w597, "命令"=w593, "板号"=w595, "命令序号"=w594, "输入数据"=w596) -> ("错误输出"=w592:errorcluster)  [unwired: 1 in, 11 out]
                        n420 = call <vilib>:"Clear Errors.vi"("error in (no error)"=w592) -> ()  [unwired: 6 in, 1 out]
                      }
                    }
                  }
                  frame #2 {
                    n421 = while {
                      tunnel: [w602] -> w600
                      i -> [w607]
                      stop <- w604 stop-if-true
                      n422 = global read "EV05全局变量1.vi" "读取超时"() -> (w602:bool)
                      n423 = local read "强制停止"() -> (w601:bool)
                      n424 = Greater Or Equal?(x=w607, y=25) -> (x >= y?=w605:bool)
                      n425 = Wait Until Next ms Multiple(millisecond multiple=u32 100 ("毫秒倍数")) -> ()  [unwired: 1 out]
                      n426 = Compound Arithmetic op=OR(w601, w602, w605) -> (w604:bool)
                    }
                  }
                  frame #3 {
                    n427 = call <vilib>:"Unset Busy.vi"() -> ()  [unwired: 2 in, 10 out]
                    n428 = case shown="假" w609 {
                      tunnel: w608 -> [w610 _]
                      frame False {
                        n429 = control-ref of="结果"() -> (w614:refnum<vi>)
                        n430 = Concatenate Strings(w610, "       写入失败" ("字符串")) -> (w613:string)
                        n431 = Build Array(w613) -> (w612:string[])
                        n432 = call "表格编辑.vi"("新元素/子数组"=w612, "活动单元格:单元格背景色"=u32 16740749, "MCListbox引用句柄"=w614) -> ()  [unwired: 9 out]
                      }
                      frame True {
                      }
                    }
                  }
                  frame #4 {
                    n433 = Increment(x=w620) -> (x+1=w616:i32)
                    n434 = Equal?(x=w621, y=w616) -> (x = y?=w619:bool)
                    n435 = And(x=w618, y=w619) -> (x .and. y?=w617:bool)
                    n436 = case shown="真" w617 {
                      frame False {
                      }
                      frame True {
                        n437 = control-ref of="结果"() -> (w625:refnum<vi>)
                        n438 = Concatenate Strings("写入完成" ("字符串")) -> (w624:string)
                        n439 = Build Array(w624) -> (w623:string[])
                        n440 = call "表格编辑.vi"("新元素/子数组"=w623, "活动单元格:单元格背景色"=u32 21937, "MCListbox引用句柄"=w625) -> ()  [unwired: 9 out]
                      }
                    }
                  }
                }
              }
              n441 = local read "强制停止"() -> (w512:bool)
              n442 = Or(x=w510, y=w512) -> (x .or. y?=w511:bool)
            }
            n443 = stacked-sequence {
              tunnel: w502 -> [_]
              frame #0 {
                n444 = local write "强制停止"(FALSE ("强制停止")) -> ()
              }
            }
          }
          frame "单个读取" {
            n445 = stacked-sequence {
              tunnel: [w657] -> w655
              frame #0 {
                n446 = local read "主从选择"() -> (w658:enum32{"主板", "从板"})
                n447 = case shown="\"主板\", 默认" w658 {
                  tunnel: [w671 w751] -> w660
                  tunnel: [w670 w752] -> w665
                  tunnel: [0 ("从板号") w748] -> w664
                  tunnel: [0 ("板号") u8 0 ("板号")] -> w663
                  tunnel: [w666 w747] -> w661
                  frame "主板", Default {
                    n448 = local read "主板选项"() -> (w667:string)
                    n449 = case shown="\"项目信息\"" w667 {
                      tunnel: [_ u8[] [1, 2, 3, 4, 5, 6, 13, 8, 7, 9, 10, 11, 12] u8[] [1] u8[] [1] u8[] [2] u8[] [3] u8[] [4] u8[] [5] u8[] [6] u8[] [13] u8[] [7] u8[] [8] u8[] [9] u8[] [10] u8[] [14] u8[] [11] u8[] [12] u8[] [2] u8[] [3] u8[] [1] u8[] [2] u8[] [1] u8[] [2] u8[] [3] u8[] [4] u8[] [1, 2, 3, 4]] -> w671
                      tunnel: [_ u8 128 ("命令") u8 129 ("命令") u8 128 ("命令") u8 128 ("命令") u8 128 ("命令") u8 128 ("命令") u8 128 ("命令") u8 128 ("命令") u8 128 ("命令") u8 128 ("命令") u8 128 ("命令") u8 128 ("命令") u8 128 ("命令") u8 128 ("命令") u8 128 ("命令") u8 128 ("命令") u8 129 ("命令") u8 129 ("命令") u8 130 ("命令") u8 130 ("命令") u8 132 ("命令") u8 132 ("命令") u8 132 ("命令") u8 132 ("命令") u8 132 ("命令")] -> w670
                      tunnel: [_ string[] ["产品编号", "电压个数", "通道电压数", "电压起始值", "温度个数", "温度起始值", "保险位置", "电池额定实际容量", "SOC", "配置文件版本", "参数修改记录", "车牌号", "SOH"] string[] ["一级故障阀值"] string[] ["产品编号"] string[] ["电压个数"] string[] ["通道电压数"] string[] ["电压起始值"] string[] ["温度个数"] string[] ["温度起始值"] string[] ["保险位置"] string[] ["SOC"] string[] ["电池额定实际容量"] string[] ["配置文件版本"] string[] ["参数修改记录"] string[] ["校正时钟"] string[] ["车牌号"] string[] ["SOH"] string[] ["二级故障阀值"] string[] ["三级故障阀值"] string[] ["加热控制参数"] string[] ["充电控制参数"] string[] ["电池信息1"] string[] ["电池包组号"] string[] ["充放电安时"] string[] ["电池充放电次数"] string[] ["电池信息1", "电池包组号", "充放电安时", "电池充放电次数"]] -> w666
                      frame "假", Default {
                      }
                      frame "项目信息" {
                      }
                      frame "SOC过低", "SOC过高", "SOH过低", "充电电流过高", "单体电压过低", "单体电压过高", "单组电压不均衡", "单组温度不均衡", "放电电流过高", "极柱温度过高", "内阻过大", "温度过低", "温度过高", "一级故障阀值", "整组电压不均衡", "整组温度不均衡", "总电压过低", "总电压过高" {
                      }
                      frame "产品编号" {
                      }
                      frame "电压个数" {
                      }
                      frame "通道电压数" {
                      }
                      frame "电压起始值" {
                      }
                      frame "温度个数" {
                      }
                      frame "温度起始值" {
                      }
                      frame "保险位置" {
                      }
                      frame "SOC" {
                      }
                      frame "电池额定实际容量" {
                      }
                      frame "配置文件版本" {
                      }
                      frame "参数修改记录" {
                      }
                      frame "校正时钟" {
                      }
                      frame "车牌号" {
                      }
                      frame "SOH" {
                      }
                      frame "SOC过低(2)", "SOC过高(2)", "SOH过低(2)", "充电电流过高(2)", "单体电压过低(2)", "单体电压过高(2)", "单组电压不均衡(2)", "单组温度不均衡(2)", "二级故障阀值", "放电电流过高(2)", "极柱温度过高(2)", "内阻过大(2)", "温度过低(2)", "温度过高(2)", "整组电压不均衡(2)", "整组温度不均衡(2)", "总电压过低(2)", "总电压过高(2)" {
                      }
                      frame "SOC过低(3)", "SOC过高(3)", "SOH过低(3)", "充电电流过高(3)", "单体电压过低(3)", "单体电压过高(3)", "单组电压不均衡(3)", "单组温度不均衡(3)", "放电电流过高(3)", "极柱温度过高(3)", "内阻过大(3)", "三级故障阀值", "温度过低(3)", "温度过高(3)", "整组电压不均衡(3)", "整组温度不均衡(3)", "总电压过低(3)", "总电压过高(3)" {
                      }
                      frame "风机关闭温差", "风机关闭温度", "风机开启温差", "风机开启温度", "加热关闭温差", "加热关闭温度", "加热开启温度", "加热控制参数" {
                      }
                      frame "充电控制参数", "电流步长", "最大允许充电电流", "最大允许充电温度", "最大允许单体电压", "最大允许总电压", "最小允许充电电流", "最小允许充电温度", "最小允许单体电压" {
                      }
                      frame "电池信息1" {
                      }
                      frame "电池包组号" {
                      }
                      frame "充放电安时" {
                      }
                      frame "电池充放电次数" {
                      }
                      frame "电池信息" {
                      }
                    }
                  }
                  frame "从板" {
                    n450 = local read "从板选项"() -> (w749:string)
                    n451 = case shown="\"SOC过低(2)\", \"电压不均衡(2)\", \"电压过低(2)\", \"电压过高(2)\", \"二级故障阀值\", \"温度不均衡(2)\", \"温度过低(2)\", \"温度过高(2)\"" w749 {
                      tunnel: [_ u8 0 ("命令") u8 0 ("命令") u8 0 ("命令") u8 0 ("命令") u8 0 ("命令") u8 0 ("命令") u8 0 ("命令") u8 2 ("命令") u8 2 ("命令") u8 2 ("命令") u8 3 ("命令") u8 3 ("命令") u8 3 ("命令") u8 3 ("命令") u8 3 ("命令") u8 3 ("命令") u8 3 ("命令") u8 3 ("命令")] -> w752
                      tunnel: [_ u8[] [6] u8[] [6, 1, 2, 3, 4, 5] u8[] [1] u8[] [2] u8[] [3] u8[] [4] u8[] [5] u8[] [1] u8[] [2] u8[] [3] u8[] [1, 2, 3, 4, 5, 6, 7] u8[] [1] u8[] [2] u8[] [3] u8[] [4] u8[] [5] u8[] [6] u8[] [7]] -> w751
                      tunnel: [_ string[] ["从板号"] string[] ["从板号", "电压起始值", "通道电压个数", "保险位置", "温度起始值", "加热控制参数"] string[] ["电压起始值"] string[] ["通道电压节数"] string[] ["保险位置"] string[] ["温度起始值"] string[] ["加热控制参数"] string[] ["一级故障阀值"] string[] ["二级故障阀值"] string[] ["三级故障阀值"] string[] ["电池包信息1", "电池包序号", "充放电安时", "充电次数时间", "SOC", "车牌号", "充电参数"] string[] ["电池包信息1"] string[] ["电池包序号"] string[] ["充放电安时"] string[] ["充电次数时间"] string[] ["SOC"] string[] ["车牌号"] string[] ["充电参数"]] -> w747
                      frame "假", Default {
                      }
                      frame "从板号" {
                      }
                      frame "从板信息" {
                      }
                      frame "电压起始值" {
                      }
                      frame "通道电压节数" {
                      }
                      frame "保险位置" {
                      }
                      frame "温度起始值" {
                      }
                      frame "风机关闭温差", "风机关闭温度", "风机开启温差", "风机开启温度", "加热关闭温差", "加热关闭温度", "加热开启温度", "加热控制参数" {
                      }
                      frame "SOC过低", "电压不均衡", "电压过低", "电压过高", "温度不均衡", "温度过低", "温度过高", "一级故障阀值" {
                      }
                      frame "SOC过低(2)", "电压不均衡(2)", "电压过低(2)", "电压过高(2)", "二级故障阀值", "温度不均衡(2)", "温度过低(2)", "温度过高(2)" {
                      }
                      frame "SOC过低(3)", "电压不均衡(3)", "电压过低(3)", "电压过高(3)", "三级故障阀值", "温度不均衡(3)", "温度过低(3)", "温度过高(3)" {
                      }
                      frame "快换参数" {
                      }
                      frame "电池包信息1" {
                      }
                      frame "电池包序号" {
                      }
                      frame "充放电安时" {
                      }
                      frame "充电次数时间" {
                      }
                      frame "SOC" {
                      }
                      frame "车牌号" {
                      }
                      frame "充电参数" {
                      }
                    }
                    n452 = local read "从板板号"() -> (w748:u8)
                  }
                }
                n453 = Build Array(w663) -> (w662:i32[])
                n454 = local write "命令"(w665) -> ()
                n455 = Array Size(array=w660) -> (size(s)=w659:i32)
                n456 = for {
                  tunnel: w660 -> [w815] mode=indexing
                  tunnel: w665 -> [w814]
                  tunnel: w664 -> [w813]
                  tunnel: w662 -> [w812]
                  tunnel: w661 -> [w811] mode=indexing
                  tunnel: w659 -> [w810]
                  tunnel: w658 -> [w808]
                  tunnel: [w807] -> w657
                  i -> [w809]
                  n457 = while {
                    tunnel: w815 -> [w824]
                    tunnel: w814 -> [w823]
                    tunnel: w813 -> [w822]
                    tunnel: w812 -> [w821]
                    tunnel: w811 -> [w820]
                    tunnel: w810 -> [w819]
                    tunnel: w809 -> [w818]
                    tunnel: w808 -> [w817]
                    tunnel: [w816] -> w807
                    stop <- w816 stop-if-true
                    n458 = stacked-sequence {
                      seq-local: [_ _ _ w974 _ _] -> [_ _ _ _ w983 _]
                      tunnel: w824 -> [_ _ w958 _ _ _]
                      tunnel: w823 -> [_ _ w957 _ _ _]
                      tunnel: w822 -> [_ _ w956 _ _ _]
                      tunnel: w821 -> [_ _ w955 _ _ _]
                      tunnel: [_ _ _ w975 _ _] -> w816
                      tunnel: w820 -> [w826 _ _ _ w984 _]
                      tunnel: w819 -> [_ _ _ _ _ w994]
                      tunnel: w818 -> [_ _ _ _ _ w993]
                      tunnel: w817 -> [w825 _ _ _ _ _]
                      frame #0 {
                        n459 = case shown="\"主板\", 默认" w825 {
                          tunnel: w826 -> [w827 w919]
                          frame "主板", Default {
                            n460 = case shown="\"参数修改记录\"" w827 {
                              frame "假", Default {
                              }
                              frame "产品编号" {
                                n461 = control-ref of="产品编号"() -> (w829:refnum<vi>)
                                n462 = property class="Str"(reference=w829, "Value"="") -> ()  [unwired: 1 in, 2 out]
                              }
                              frame "电压个数" {
                                n463 = local read "从板个数"() -> (w835:dbl)
                                n464 = control-ref of="项目信息"() -> (w833:refnum<vi>)
                                n465 = Increment(x=w835) -> (x+1=w834:dbl)
                                n466 = for {
                                N: w834 -> [_]
                                tunnel: [""] -> w832 mode=indexing
                                }
                                n467 = call "表格数据输入-8.6.vi"("行数"=u32 0, "列数"=u32 1, "字符串数组"=w832, "表格引用"=w833) -> ()  [unwired: 8 in]
                              }
                              frame "通道电压数" {
                                n468 = control-ref of="项目信息"() -> (w841:refnum<vi>)
